vi "Set Data Logging Rate.vi"   [LabVIEW 2020, in "NI_VS Data Logging API.lvlib"]
doc: "Specifies the rate at which to log data, in hertz. You can log at the rate at which the target produces data, or a custom rate. You must manually select the polymorphic instance to use."
uses:
  <vilib>/NI VeriStand/Execution/DataLogging/NI_VS Data Logging API.lvlib
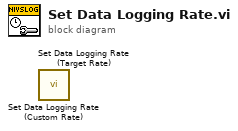
[diagram p0: block diagram]
diagram:
  n1 = call <vilib>:"Set Data Logging Rate (Custom Rate).vi"() -> ()  [unwired: 10 in, 2 out]
  n2 = call <vilib>:"Set Data Logging Rate (Target Rate).vi"() -> ()  [unwired: 10 in, 2 out]
